vi "foldersfiles.vi"(4 "error in":errorcluster, 5 "folder names":string[](array[string]), 6 "filenames":string[](array[string]), 7 "path":path) -> (0 "error out":errorcluster, 1 "Array 2":path[](array[path]), 2 "Array":T1(array[cluster]), 3 "path out":path)   [LabVIEW 2010]
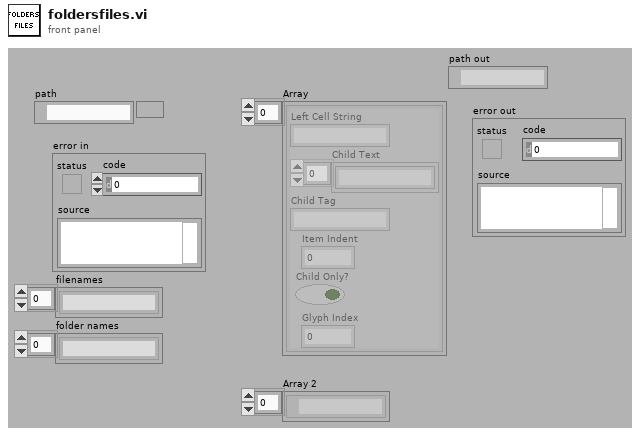
[diagram p1: front panel]
types:
  T1 = cluster{"Left Cell String":string, "Child Text":string[], "Child Tag":string, "Item Indent":i32, "Child Only?":bool, "Glyph Index":i32}[]
  T2 = cluster{"Left Cell String":string, "Child Text":string[], "Child Tag":string, "Item Indent":i32, "Child Only?":bool, "Glyph Index":i32}
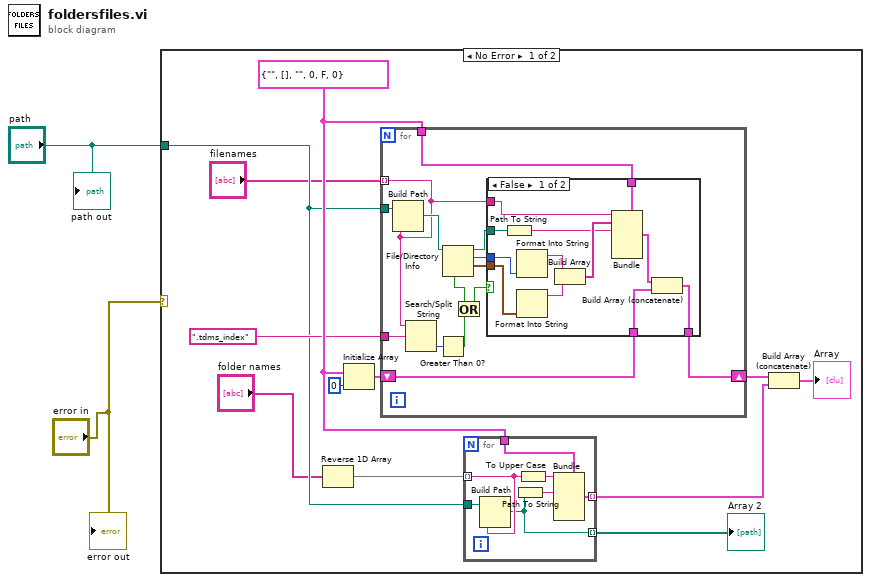
[diagram p0: block diagram]
diagram:
  n1 = case shown="No Error" "error in" {
    tunnel: "path" -> [w5 _]
    frame No Error {
      w9 = T2 {"Left Cell String"="", "Child Text"=[], "Child Tag"="", "Item Indent"=0, "Child Only?"=FALSE, "Glyph Index"=0} ("Item")
      n2 = Reverse 1D Array(array="folder names") -> (reversed array=w11:string[])
      n3 = Initialize Array(w9, 0 ("dimension size")) -> (w10:T1)
      n4 = for {
        tunnel: w9 -> [w25]
        tunnel: "filenames" -> [w22] mode=indexing
        tunnel: w5 -> [w28]
        shift-right: [w15] -> w6
        shift-left: w10 -> [w16]
        tunnel: ".tdms_index" -> [w21]
        n5 = Build Path(base path=w28, name or relative path=w22) -> (appended path=w23:path)
        n6 = Search/Split String(string=w22, search string/char (-)=w21) -> (offset of match=w20:i32)  [unwired: 1 in, 2 out]
        n7 = Greater Than 0?(x=w20) -> (x > 0?=w19:bool)
        n8 = File/Directory Info(path=w23) -> (path out=w24:path, size=w26:i64, last mod=w27:timestamp, shortcut=w18:bool)  [unwired: 1 in, 3 out]
        n9 = Or(x=w18, y=w19) -> (x .or. y?=w17:bool)
        n10 = case shown="False" w17 {
          tunnel: w27 -> [w39 _]
          tunnel: w26 -> [w40 _]
          tunnel: w25 -> [w36 _]
          tunnel: w22 -> [w34 _]
          tunnel: w24 -> [w33 _]
          tunnel: w16 -> [w30 w41]
          tunnel: [w29 w41] -> w15
          frame False {
            n11 = Path To String(path=w33) -> (string=w32:string)
            n12 = Format Into String(w40) -> (resulting string=w37:string)  [unwired: 3 in, 1 out]
            n13 = Format Into String(w39) -> (resulting string=w38:string)  [unwired: 3 in, 1 out]
            n14 = Build Array(w37, w38) -> (w35:string[])
            n15 = Bundle(cluster=w36, "Left Cell String"=w34, "Child Text"=w35, "Child Tag"=w32) -> (w31:T2)  [unwired: 3 in]
            n16 = Build Array (concatenate)(w31, w30) -> (w29:T1)
          }
          frame True {
          }
        }
      }
      n17 = for {
        tunnel: w9 -> [w48]
        tunnel: w11 -> [w46] mode=indexing
        tunnel: w5 -> [w47]
        tunnel: [w45] -> w12 mode=indexing
        tunnel: [w43] -> w13 mode=indexing
        n18 = Build Path(base path=w47, name or relative path=w46) -> (appended path=w43:path)
        n19 = Path To String(path=w43) -> (string=w44:string)
        n20 = To Upper Case(1:w46) -> (0:w42:string)
        n21 = Bundle(cluster=w48, "Left Cell String"=w42, "Child Tag"=w44) -> (w45:T2)  [unwired: 4 in]
      }
      "Array 2" <- w13
      n22 = Build Array (concatenate)(w6, w12) -> (→"Array":T1)
    }
    frame Error {
    }
  }
  "error out" <- "error in"
  "path out" <- "path"
